vi "Set Target Position.vi"(8 "error in (no error)":errorcluster, 10 "Target Point":cluster{"x":i16, "y":i16}, 11 "HIJ Vision Display in":refnum<class "HIJ Vision Display.lvclass">) -> (0 "error out":errorcluster, 3 "HIJ Vision Display out":refnum<class "HIJ Vision Display.lvclass">)   [LabVIEW 2020, in "HIJ Vision Display.lvlib" / "HIJ Vision Display.lvclass"]
uses:
  HIJ Vision Display.lvclass
  HIJ Vision Display.lvclass/HIJ Vision Display.ctl
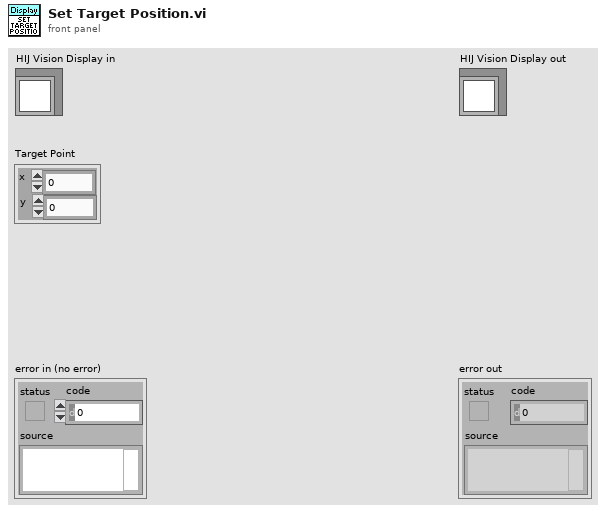
[diagram p1: front panel]
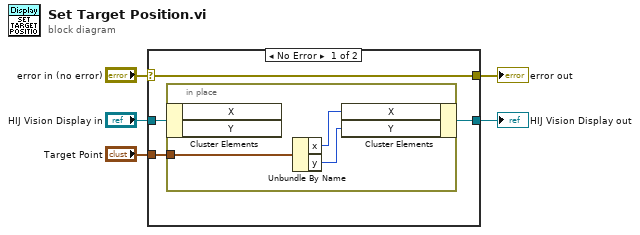
[diagram p0: block diagram]
diagram:
  n1 = case shown="No Error" "error in (no error)" {
    selector: "error in (no error)" -> [w9 w14]
    tunnel: [w9 w14] -> w4
    tunnel: [w6 w13] -> w2
    tunnel: "HIJ Vision Display in" -> [w8 w13]
    tunnel: "Target Point" -> [w7 _]
    frame No Error {
      n2 = in-place {
        in-place-border: w7 -> [w12]
        n3 = in-place-cluster #1(w8) -> ()  [unwired: 2 out]
        n4 = Unbundle By Name(w12) -> ("x"=w11:i16, "y"=w10:i16)
        n5 = in-place-cluster #1("X"=w11, "Y"=w10) -> (w6:refnum<class "HIJ Vision Display.lvclass">)
      }
    }
    frame Error {
    }
  }
  "error out" <- w4
  "HIJ Vision Display out" <- w2
